vi "Get PanelVIPath.vi"(6 "error in (no error)":errorcluster caption="错误输入（无错误）", 8 "Split Mode":T1, 9 "PanelDataNode 输入":refnum<class "PanelDataNode.lvclass"> caption="DNL_LabVIEW Object in") -> (0 "error out":errorcluster caption="错误输出", 2 "panel path":path, 3 "PanelDataNode 输出":refnum<class "PanelDataNode.lvclass"> caption="DNL_LabVIEW Object out")   [LabVIEW 2016, in "PanelDataNode.lvclass"]
uses:
  PanelDataNode.lvclass
  Split Mode.ctl
  PanelDataNode.lvclass/PanelDataNode.ctl
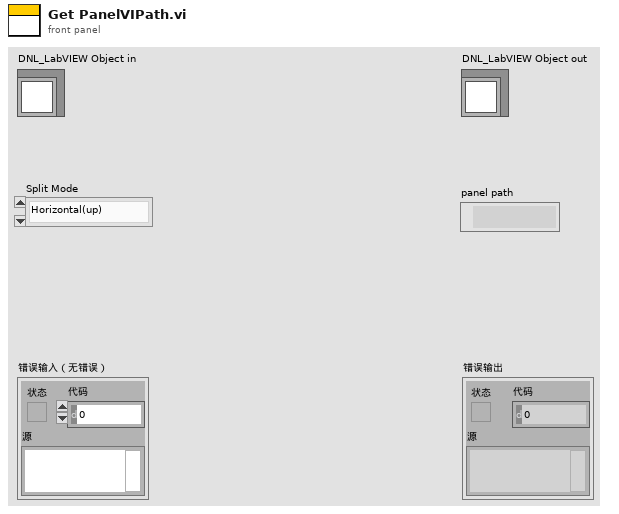
[diagram p1: front panel]
types:
  T1 = typedef "PanelDataNode.lvclass/Split Mode.ctl" = enum16{"Horizontal(up)", "Vertical(left)", "Horizontal(down)", "Vertical(right)"}
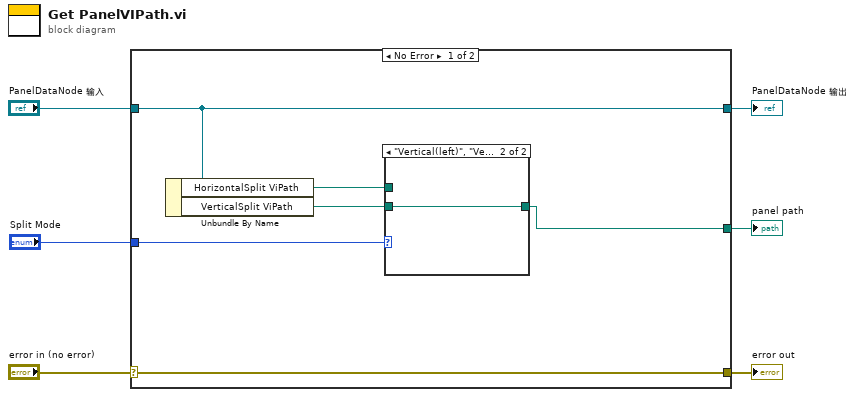
[diagram p0: block diagram]
diagram:
  n1 = case shown="No Error" "error in (no error)" {
    selector: "error in (no error)" -> [w7 w16]
    tunnel: [w7 w16] -> w5
    tunnel: [w11 w15] -> w3
    tunnel: "PanelDataNode 输入" -> [w11 w15]
    tunnel: "Split Mode" -> [w12 _]
    tunnel: [w8 _] -> w1
    frame No Error {
      n2 = Unbundle By Name(w11) -> ("HorizontalSplit ViPath"=w10:path, "VerticalSplit ViPath"=w9:path)
      n3 = case shown="\"Vertical(left)\", \"Vertical(right)\"" w12 {
        tunnel: w10 -> [w13 _]
        tunnel: w9 -> [_ w14]
        tunnel: [w13 w14] -> w8
        frame "Horizontal(up)", "Horizontal(down)" {
        }
        frame "Vertical(left)", "Vertical(right)" {
        }
      }
    }
    frame Error {
    }
  }
  "error out" <- w5
  "PanelDataNode 输出" <- w3
  "panel path" <- w1
